vi "LEP_RV_Explore.vi"   [LabVIEW 2011]
types:
  T1 = typedef "LEP_RV_Config.ctl" = cluster{"Enable debugging":bool, "Debug Options":u16, "Use stack variables":bool, "Generate serial only":bool, "Generate guard code":bool, "Generate Integer Only":bool, "Generate C Function Calls":bool, "ExpressionFolding":bool, "Constant Allocation":u16, "Constant Deallocation":u16, "Build Specification ID":string, "Preprocessor symbols (define)":string, "Compiler Flags":string, "Linker Flags":string, "Mode":u16, "Optimization":u16, "Optimize for time":bool, "Enable cross-module optimization":bool, "Include paths":path[], "Optimize heap size":bool, "Use MicroLib":bool, "Debug Mode":u16, "Enable profile information":bool, "Host name":string, "Use DHCP":bool, "IP address":string, "Subnet mask":string, "Gateway":string, "Primary DNS":string, "Secondary DNS":string, "MAC in target memory":bool, "MAC address":string, "Console output":u16, "Target serial port":u16}
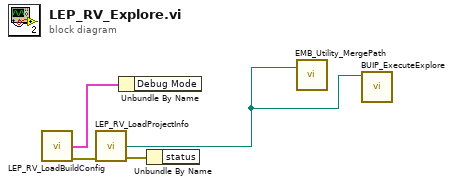
[diagram p0: block diagram]
diagram:
  n1 = call "LEP_RV_LoadBuildConfig.vi"() -> ("Config"=w3:T1, "error out"=w4:errorcluster)  [unwired: 1 in, 1 out]
  n2 = call "LEP_RV_LoadProjectInfo.vi"("error in (no error)"=w4) -> ("Build Path"=w1:path, "error out"=w2:errorcluster)  [unwired: 8 in, 5 out]
  n3 = Unbundle By Name(w3) -> ()  [unwired: 1 out]
  n4 = Unbundle By Name(w2) -> ()  [unwired: 1 out]
  n5 = call <vilib>:"EMB_Utility_MergePath.vi"("Base Path"=w1) -> ()  [unwired: 1 in, 1 out]
  n6 = call "BUIP_ExecuteExplore.vi"("PathToExplore"=w1) -> ()  [unwired: 11 in]
